vi "DoGetNewUser.vi"(7 "error in (no error)":errorcluster, 8 "LastUserName":string, 9 "IsInitialLogin":bool, 10 "Sequence Context In":refnum<k7>) -> (0 "error out":errorcluster, 1 "LoginName":string, 2 "isValidUser":bool, 3 "Sequence Context Out":refnum<k7>)   [LabVIEW 2020]
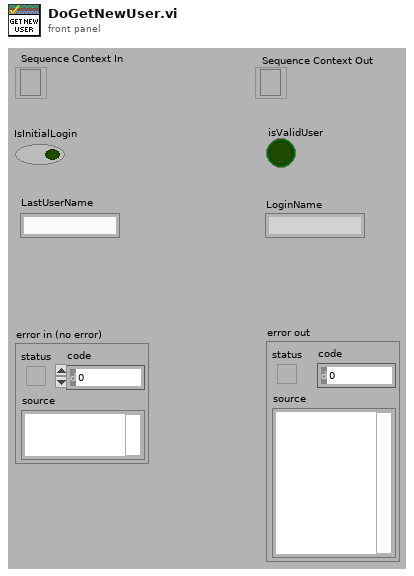
[diagram p1: front panel]
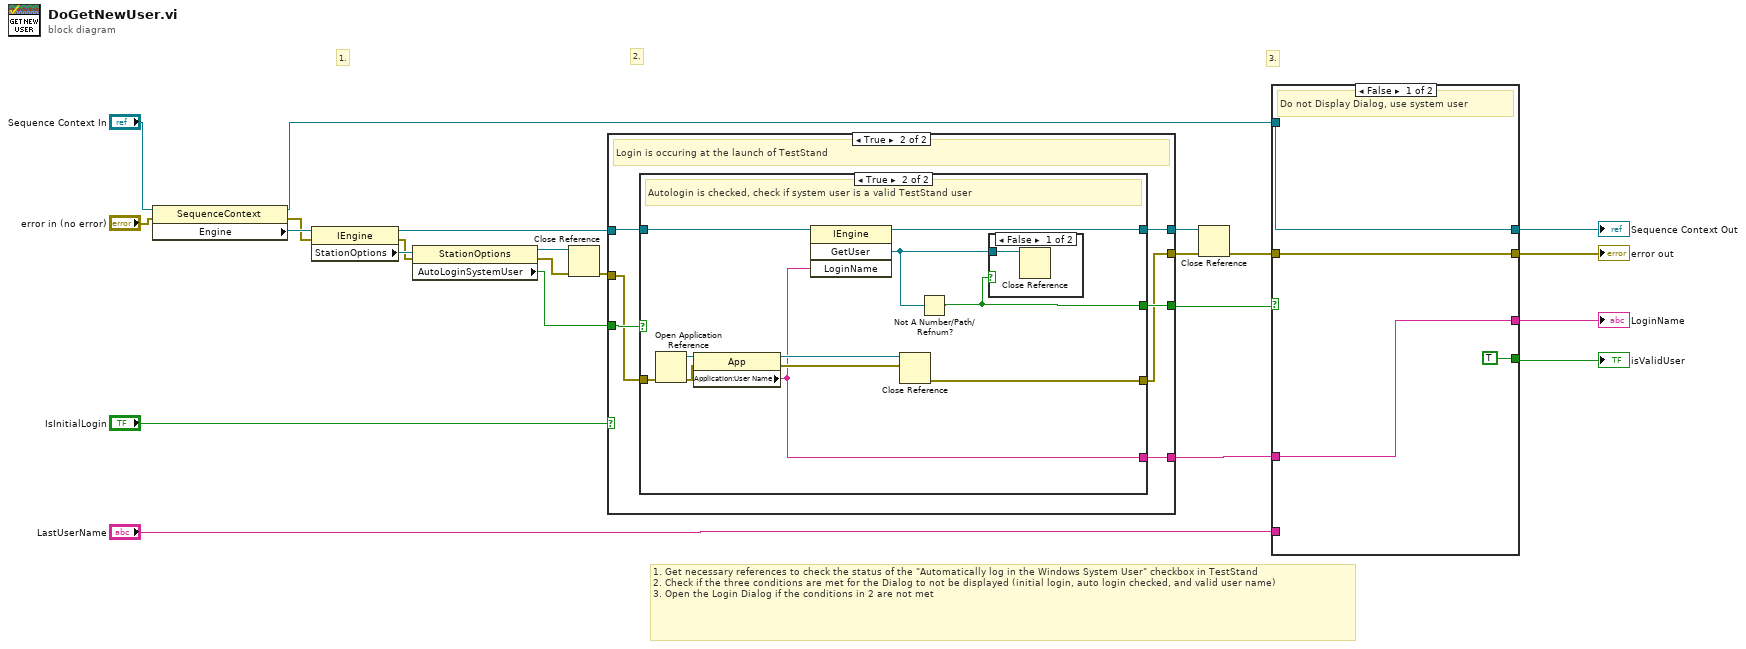
[diagram p0: block diagram]
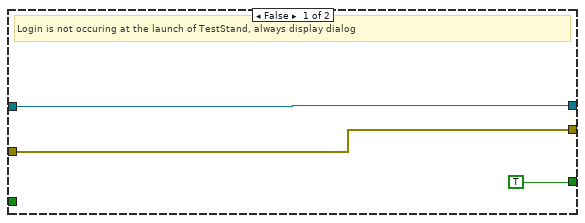
[diagram p2: hidden frame]
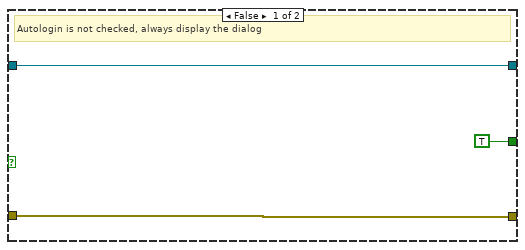
[diagram p3: hidden frame]
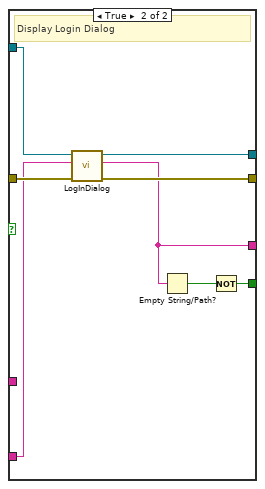
[diagram p5: hidden frame]
diagram:
  # "1. Get necessary references to check the status of the \"Automatically log in the Windows System User\" checkbox in TestStand\n2. Check if the three conditions are met for the Dialog to not be displayed (initial login, auto login checked, and valid user name)\n3. Open the Login Dialog if the conditions in 2 are not met"
  # "3."
  # "2."
  # "1."
  n1 = property class="SequenceContext"(reference="Sequence Context In", error in="error in (no error)") -> (reference out=w10:refnum<k7>, error out=w2:errorcluster, "Engine"=w16:refnum<k7>)
  n2 = property class="IEngine"(reference=w16, error in=w2) -> (reference out=w20:refnum<k7>, error out=w19:errorcluster, "StationOptions"=w23:refnum<k7>)
  n3 = property class="StationOptions"(reference=w23, error in=w19) -> (reference out=w15:refnum<k7>, error out=w13:errorcluster, "AutoLoginSystemUser"=w21:bool)
  n4 = Close Reference(reference=w15, error in (no error)=w13) -> (error out=w14:errorcluster)
  n5 = case shown="True" "IsInitialLogin" {
    tunnel: w21 -> [_ w33]
    tunnel: [TRUE ("displayLoginDialog") w32] -> w17
    tunnel: w20 -> [w24 w29]
    tunnel: [w25 w30] -> w8
    tunnel: w14 -> [w25 w31]
    tunnel: [w24 w28] -> w6
    tunnel: [_ w27] -> w1
    frame False {
      # "Login is not occuring at the launch of TestStand, always display dialog"
    }
    frame True {
      # "Login is occuring at the launch of TestStand"
      n6 = case shown="True" w33 {
        tunnel: [TRUE ("displayLoginDialog") w37] -> w32
        tunnel: w31 -> [w35 w47]
        tunnel: [w35 w44] -> w30
        tunnel: w29 -> [w34 w41]
        tunnel: [w34 w40] -> w28
        tunnel: [_ w39] -> w27
        frame False {
          # "Autologin is not checked, always display the dialog"
        }
        frame True {
          # "Autologin is checked, check if system user is a valid TestStand user"
          n7 = Open Application Reference(8:w47) -> (0:w45:errorcluster, 3:w46:refnum<vi>)  [unwired: 3 in]
          n8 = property class="App"(reference=w46, error in=w45) -> (reference out=w43:refnum<vi>, error out=w42:errorcluster, "Application:User Name"=w39:string)
          n9 = invoke class="IEngine" method="GetUser"(reference=w41, "LoginName"=w39) -> (reference out=w40:refnum<k7>, "GetUser"=w38:refnum<k7>)  [unwired: 2 in, 2 out]
          n10 = Close Reference(reference=w43, error in (no error)=w42) -> (error out=w44:errorcluster)
          n11 = Not A Number/Path/Refnum?(number/path/refnum=w38) -> (NaN/Path/Refnum?=w37:bool)
          n12 = case shown="False" w37 {
            tunnel: w38 -> [w48 _]
            frame False {
              n13 = Close Reference(reference=w48) -> ()  [unwired: 1 in, 1 out]
            }
            frame True {
            }
          }
        }
      }
    }
  }
  n14 = Close Reference(reference=w6, error in (no error)=w8) -> (error out=w7:errorcluster)
  n15 = case shown="False" w17 {
    tunnel: [w50 w58] -> w5
    tunnel: [TRUE ("HasPrivilege") w53] -> w18
    tunnel: [w49 w55] -> w9
    tunnel: "LastUserName" -> [_ w56]
    tunnel: w10 -> [w51 w60]
    tunnel: [w51 w59] -> w11
    tunnel: w7 -> [w50 w57]
    tunnel: w1 -> [w49 _]
    frame False {
      # "Do not Display Dialog, use system user"
    }
    frame True {
      # "Display Login Dialog"
      n16 = call "LogInDialog.vi"("error in (no error)"=w57, "Default User"=w56, "Sequence Context In"=w60) -> ("error out"=w58:errorcluster, "UserName"=w55:string, "Sequence Context Out"=w59:refnum<k7>)  [unwired: 6 in]
      n17 = Empty String/Path?(string/path=w55) -> (empty?=w54:bool)
      n18 = Not(x=w54) -> (.not. x?=w53:bool)
    }
  }
  "error out" <- w5
  "isValidUser" <- w18
  "LoginName" <- w9
  "Sequence Context Out" <- w11
